vi "Core Actor (ROOT) - Dispatch Message to Child (Nested_Actor).vi"(8 "error in (no error)":errorcluster, 11 "Child_3_Class in":refnum<class "SW_Interface_Class.lvclass">) -> (0 "error out":errorcluster, 3 "Child_3_Class out":refnum<class "SW_Interface_Class.lvclass">)   [LabVIEW 2023, in "SW_Interface_Actor.lvlib" / "SW_Interface_Class.lvclass"]
uses:
  SW_Interface_Class.lvclass
  SW_Interface_Class.lvclass/SW_Interface_Class.ctl
  SW_Interface_Class Messages/Core Actor - Send Actor Message Msg/Core Actor - Send Actor Message Msg.lvclass/Core Actor - Send Actor Message Msg.ctl
  <vilib>/ActorFramework/Message Enqueuer/Message Enqueuer.lvclass/Message Enqueuer.ctl
  <vilib>/ActorFramework/Message Enqueuer/Enqueue.vi
  SW_Interface_Class Messages/Core Actor - Send Actor Message Msg/Core Actor - Send Actor Message Msg.lvclass
  Applications/National Instruments/LabVIEW 2023 64-bit/vi.lib/ActorFramework/Message/Message.lvclass
  <vilib>/ActorFramework/Message Priority Queue/Priority Enqueue.vi
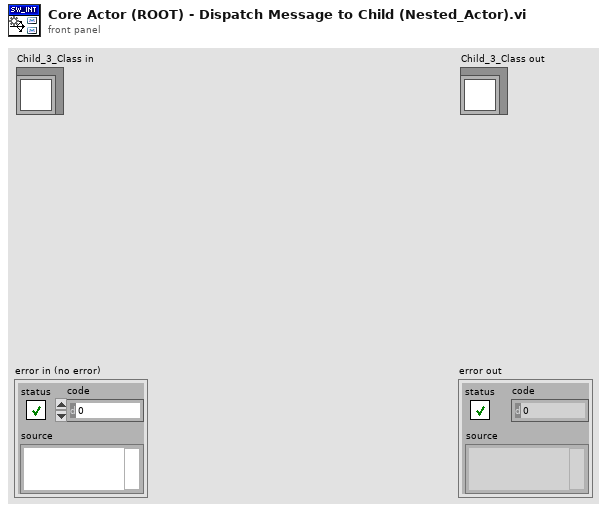
[diagram p1: front panel]
types:
  T1 = typedef "SW_Interface_Actor.lvlib/SW_Interface_Class.lvclass/SW Interface - Ctrl - Trigger Event Cluster.ctl" = cluster{"Events":T2, "Data":string}
  T2 = typedef "SW_Interface_Actor.lvlib/SW_Interface_Class.lvclass/SW Interface - Ctrl - Enum - Events (Temp).ctl" = enum16{"SEND MESSAGE Ev", "STOP_ACTOR Ev", "INIT_ACTOR Ev", "START Ev", "STOP Ev", "GET Ev", "SET Ev", "ERROR_HANDLER Ev", "RESET Ev", "T2 Ev", "T3 Ev", "T4 Ev"}
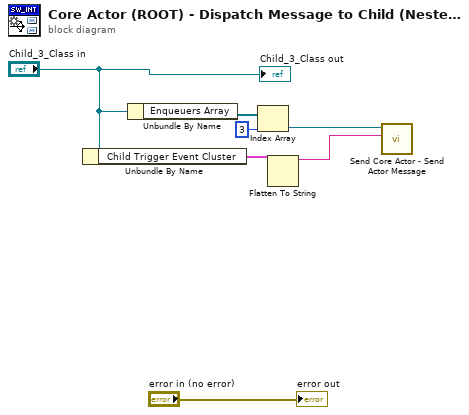
[diagram p0: block diagram]
diagram:
  n1 = Unbundle By Name("Child_3_Class in") -> ("Child Trigger Event Cluster"=w3:T1)
  n2 = Unbundle By Name("Child_3_Class in") -> ("Enqueuers Array"=w6:refnum<class "Message Enqueuer.lvclass">[])
  n3 = Index Array(array=w6, index=3) -> (element=w2:refnum<class "Message Enqueuer.lvclass">)
  n4 = Flatten To String(anything=w3) -> (data string=w1:string)  [unwired: 3 in, 2 out]
  n5 = call "Send Core Actor - Send Actor Message.vi"("Value"=w1, "Message Enqueuer"=w2) -> ()  [unwired: 8 in, 2 out]
  "error out" <- "error in (no error)"
  "Child_3_Class out" <- "Child_3_Class in"
